vi "Nicht blockierende (Fehler) Meldung ablaufinvariant.vi"() -> ()   [LabVIEW 2015, in "SysLog.lvlib"]
doc: "Fehlermeldung zum Anzeigen der aktuellen Fehlermeldung aber ablaufinvariant ohne nix - für den exit case.\nLiest nur die letze Fehlermeldung aus dem zugehörigen FGV.\n#ErrLogHistory\nriw 8.6.2018"
uses:
  SysLog.lvlib
panel:
  out "Beschreibung":string
  out "Meldung":string
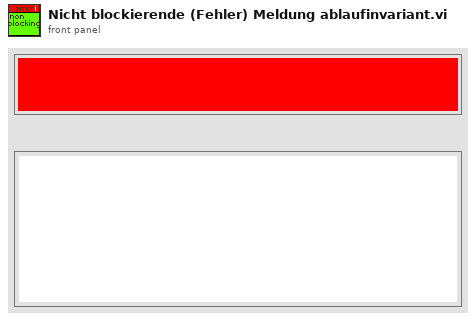
[diagram p1: front panel]
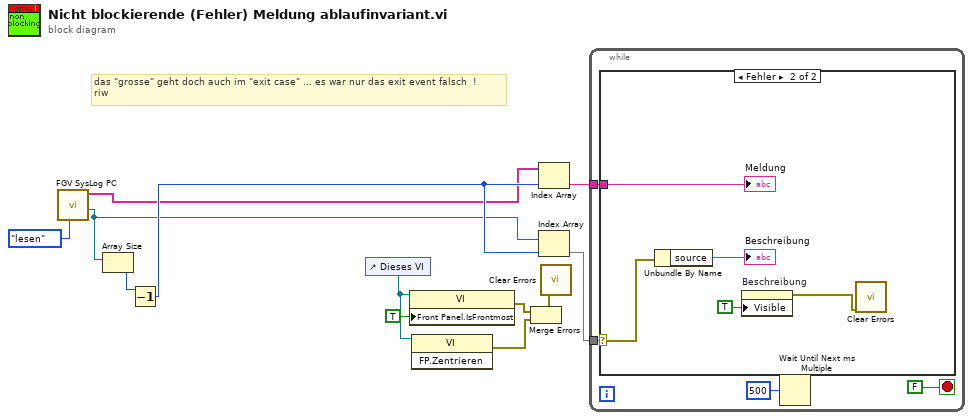
[diagram p0: block diagram]
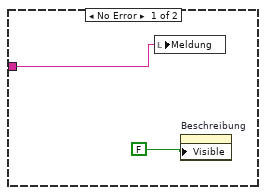
[diagram p2: hidden frame]
diagram:
  # "das \"grosse\" geht doch auch im \"exit case\" ... es war nur das exit event falsch  !\nriw"
  n1 = call "FGV SysLog PC.vi"("Aktion"=enum16{"initialisieren", "lesen", "schreiben"}."lesen") -> ("Main History Button Referenz out"=w2:refnum<vi>, "Message Array"=w1:string[])  [unwired: 5 in, 4 out]
  n2 = Array Size(array=w2) -> (size(s)=w12:i32)
  n3 = Decrement(x=w12) -> (x-1=w3:i32)
  n4 = control-ref of="Dieses VI"() -> (w6:refnum<vi>)
  n5 = property class="VI"(reference=w6, "Front Panel.IsFrontmost"=TRUE ("Frontpanel-Fenster:Ist im Vordergrund")) -> (error out=w7:errorcluster)  [unwired: 1 in, 1 out]
  n6 = invoke class="VI" method="FP.Zentrieren"(reference=w6) -> (error out=w4:errorcluster)  [unwired: 2 in, 2 out]
  n7 = Merge Errors(w7, w4) -> (w5:errorcluster)
  n8 = Index Array(array=w1, index=w3) -> (element=w10:string)
  n9 = Index Array(array=w2, index=w3) -> (element=w9)
  n10 = call <vilib>:"Clear Errors.vi"("error in (no error)"=w5) -> ()  [unwired: 5 in, 2 out]
  n11 = while {
    tunnel: w10 -> [w16]
    tunnel: w9 -> [w15]
    stop <- FALSE stop-if-true
    n12 = case shown="Fehler" w15 {
      selector: w15 -> [_ w23]
      tunnel: w16 -> [w17 w21]
      frame No Error {
        n13 = local write "Meldung"(w17) -> ()
        n14 = property on="Beschreibung" class="Str"("Visible"=FALSE ("Sichtbar")) -> ()  [unwired: 2 in, 2 out]
      }
      frame Error {
        n15 = Unbundle By Name(w23) -> ("source"=→"Beschreibung":string)
        n16 = property on="Beschreibung" class="Str"("Visible"=TRUE ("Sichtbar")) -> (error out=w19:errorcluster)  [unwired: 2 in, 1 out]
        n17 = call <vilib>:"Clear Errors.vi"("error in (no error)"=w19) -> ()  [unwired: 5 in, 2 out]
        "Meldung" <- w21
      }
    }
    n18 = Wait Until Next ms Multiple(millisecond multiple=u32 500 ("ms")) -> ()  [unwired: 1 out]
  }
